vi "zad3.vi"() -> ()   [LabVIEW 2017]
panel:
  out "Intensity Graph":dbl[][](graph)
  out "Array":dbl[][](array[numeric])
  in  "Radio Buttons":enum32{"A", "B", "C", "D"}(radio)
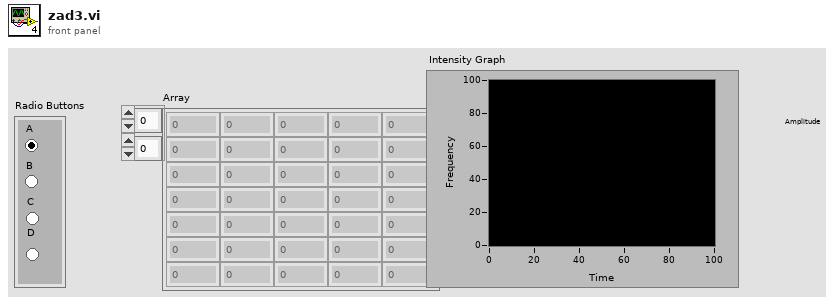
[diagram p1: front panel]
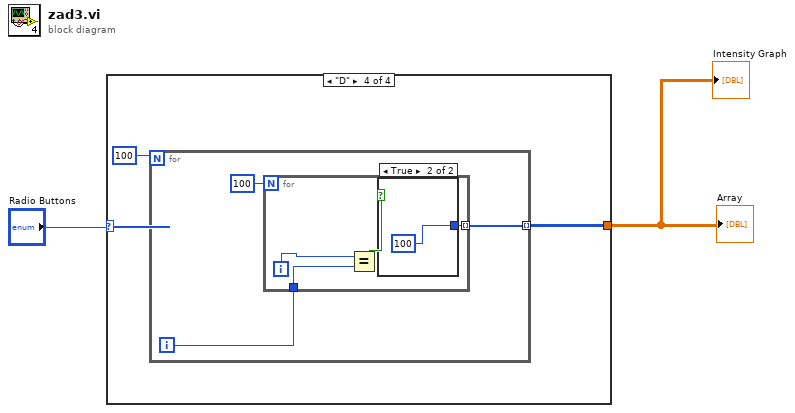
[diagram p0: block diagram]
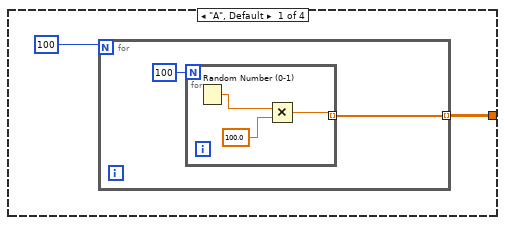
[diagram p2: hidden frame]
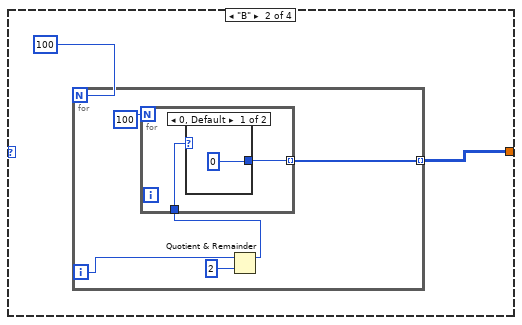
[diagram p3: hidden frame]
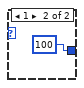
[diagram p4: hidden frame]
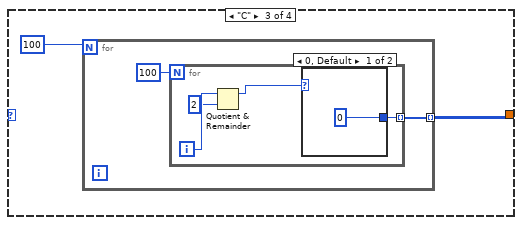
[diagram p5: hidden frame]
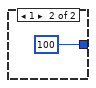
[diagram p6: hidden frame]
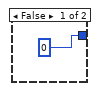
[diagram p7: hidden frame]
diagram:
  n1 = case shown="\"D\"" "Radio Buttons" {
    tunnel: [w3 w10 w21 w31] -> w1
    frame "A", Default {
      n2 = for {
        N: 100 -> [_]
        tunnel: [w5] -> w3 mode=indexing
        n3 = for {
          N: 100 -> [_]
          tunnel: [w8] -> w5 mode=indexing
          n4 = Random Number (0-1)() -> (number: 0 to 1=w9:dbl)
          n5 = Multiply(x=w9, y=100.0) -> (x*y=w8:dbl)
        }
      }
    }
    frame "B" {
      n6 = for {
        N: 100 -> [_]
        tunnel: [w12] -> w10 mode=indexing
        i -> [w15]
        n7 = Quotient & Remainder(x=w15, y=2) -> (x-y*floor(x/y)=w13:i32)  [unwired: 1 out]
        n8 = for {
          N: 100 -> [_]
          tunnel: w13 -> [w18]
          tunnel: [w17] -> w12 mode=indexing
          n9 = case shown="0, Default" w18 {
            tunnel: [0 100] -> w17
            frame 0, Default {
            }
            frame 1 {
            }
          }
        }
      }
    }
    frame "C" {
      n10 = for {
        N: 100 -> [_]
        tunnel: [w23] -> w21 mode=indexing
        n11 = for {
          N: 100 -> [_]
          tunnel: [w28] -> w23 mode=indexing
          i -> [w27]
          n12 = Quotient & Remainder(x=w27, y=2) -> (x-y*floor(x/y)=w25:i32)  [unwired: 1 out]
          n13 = case shown="0, Default" w25 {
            tunnel: [0 100] -> w28
            frame 0, Default {
            }
            frame 1 {
            }
          }
        }
      }
    }
    frame "D" {
      n14 = for {
        N: 100 -> [_]
        tunnel: [w33] -> w31 mode=indexing
        i -> [w34]
        n15 = for {
          N: 100 -> [_]
          tunnel: w34 -> [w39]
          tunnel: [w36] -> w33 mode=indexing
          i -> [w38]
          n16 = Equal?(x=w38, y=w39) -> (x = y?=w37:bool)
          n17 = case shown="True" w37 {
            tunnel: [0 100] -> w36
            frame False {
            }
            frame True {
            }
          }
        }
      }
    }
  }
  "Array" <- w1
  "Intensity Graph" <- w1
